vi "ismatec_test.vi"() -> ()   [LabVIEW 2015]
uses:
  x64/Debug/BERTTA.dll
panel:
  in  "speed":sgl
  in  "Device port":i32=15
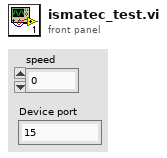
[diagram p1: front panel]
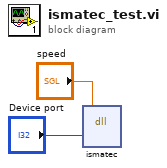
[diagram p0: block diagram]
diagram:
  n1 = dll-call lib="C:/Users/shresplab/OneDrive - Kemira Oyj/Documents/Visual Studio 2017/Projects/Bertta/BERTTA/x64/Debug/BERTTA.dll" fn="ismatec"("port"="Device port", "speed"="speed") -> ()  [unwired: 6 in, 2 out]
